vi "rename tag.vi"(7 "owner ID":string, 8 "error in":errorcluster, 9 "new name":string, 10 "old name":string, 11 "engine configuration in":refnum<class "engine configuration.lvclass">) -> (0 "error out":errorcluster, 3 "engine configuration out":refnum<class "engine configuration.lvclass">)   [LabVIEW 2013, in "engine configuration.lvclass"]
doc: "This function is used to rename a tag. If a tag claims to have an owner, only that owner is allowed to modify the tag name."
uses:
  engine configuration.lvclass
  <vilib>/NI/Tag Bus/tag/tag descriptor.lvclass
  <vilib>/NI/Tag Bus/tag/tag descriptor.lvclass/tag descriptor.ctl
  engine configuration.lvclass/engine configuration.ctl
  <vilib>/NI/Configuration Framework/NISE_CEF_TreeControl.lvlib
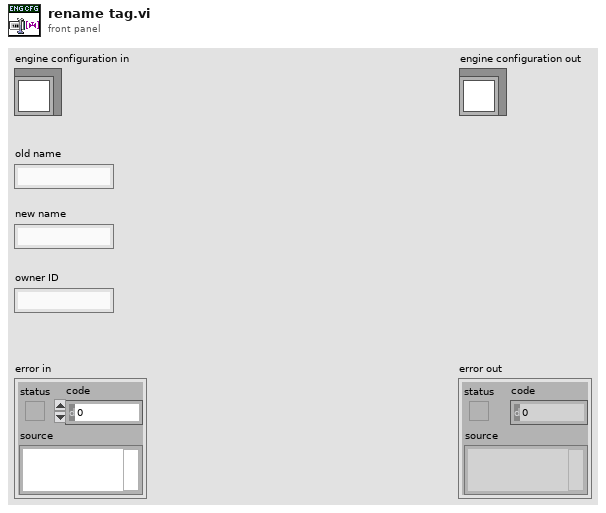
[diagram p1: front panel]
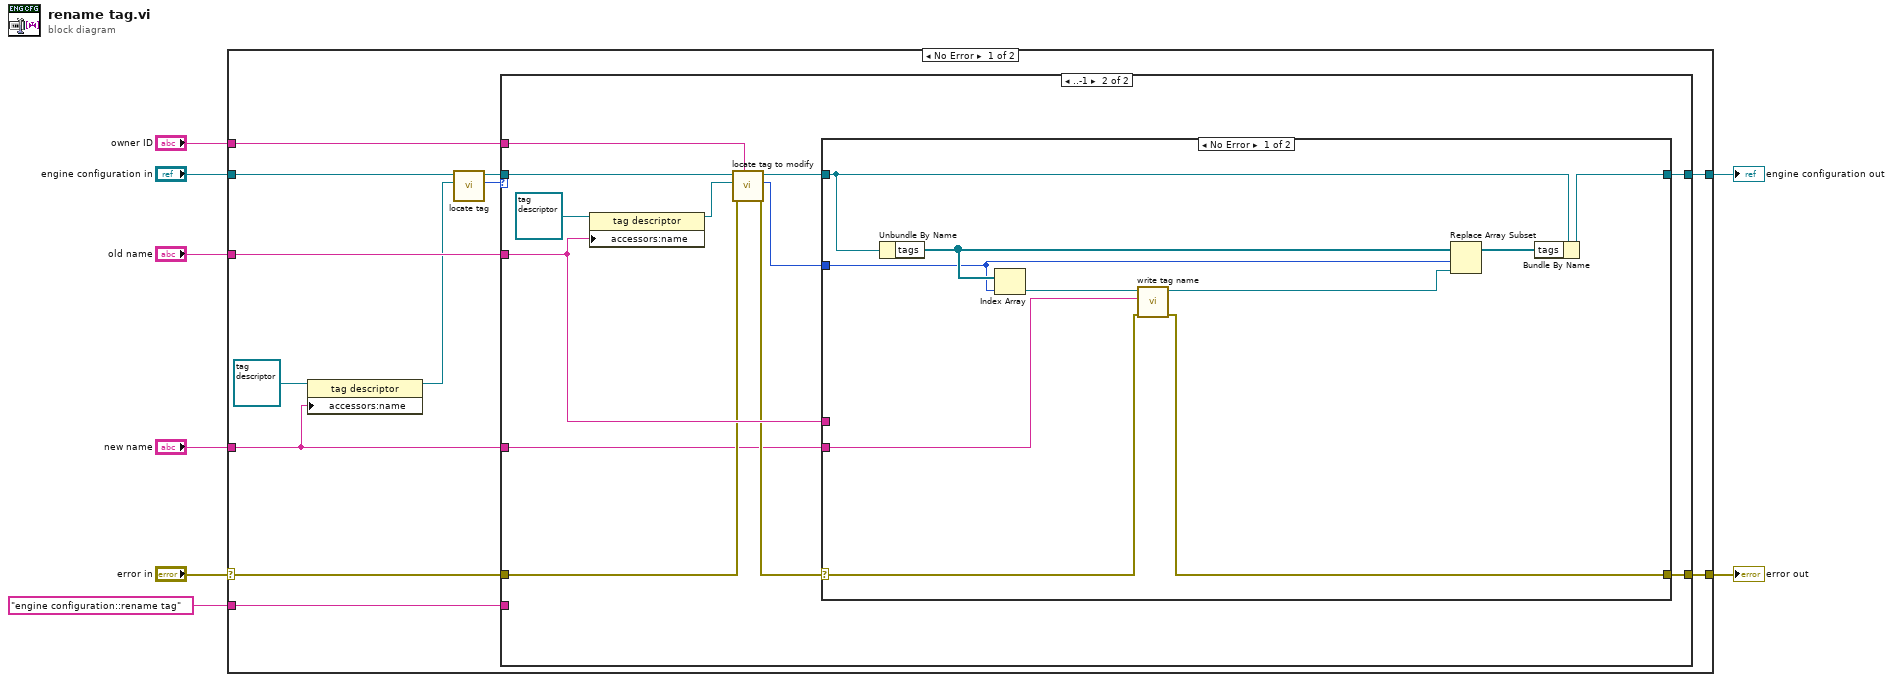
[diagram p0: block diagram]
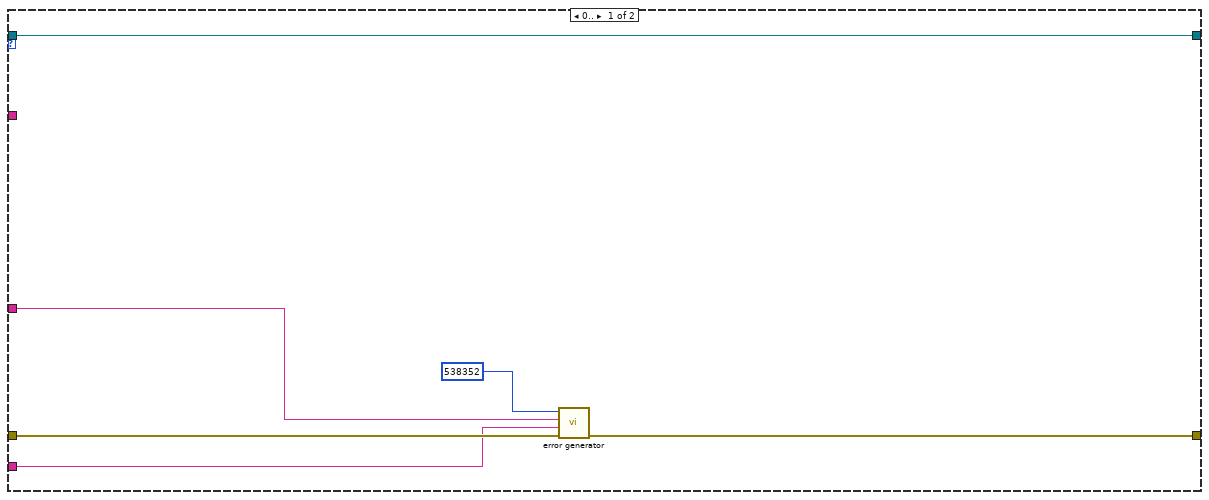
[diagram p2: hidden frame]
diagram:
  n1 = case shown="No Error" "error in" {
    selector: "error in" -> [w16 w52]
    tunnel: [w20 w52] -> w7
    tunnel: [w19 w51] -> w5
    tunnel: "engine configuration in" -> [w15 w51]
    tunnel: "old name" -> [w18 _]
    tunnel: "new name" -> [w12 _]
    tunnel: "owner ID" -> [w17 _]
    tunnel: "engine configuration::rename tag" ("source") -> [w9 _]
    frame No Error {
      n2 = property class="tag descriptor"(reference=refnum<class "tag descriptor.lvclass"> refnum ("tag descriptor"), "accessors:name"=w12) -> (reference out=w11:refnum<class "tag descriptor.lvclass">)  [unwired: 1 in, 1 out]
      n3 = call "locate tag.vi"("tag descriptor"=w11, "engine configuration in"=w15) -> ("index"=w10:i32, "engine configuration out"=w14:refnum<class "engine configuration.lvclass">)  [unwired: 8 in]
      n4 = case shown="..-1" w10 {
        tunnel: [w24 w37] -> w20
        tunnel: [w26 w36] -> w19
        tunnel: w18 -> [_ w35]
        tunnel: w17 -> [_ w33]
        tunnel: w16 -> [w25 w31]
        tunnel: w14 -> [w26 w28]
        tunnel: w12 -> [w23 w27]
        tunnel: w9 -> [w21 _]
        frame 0.. {
          n5 = call <vilib>:"error generator.vi"("error in"=w25, "source"=w21, "append error message"=w23, "error code (0)"=538352) -> ("error out"=w24:errorcluster)  [unwired: 5 in]
        }
        frame ..-1 {
          n6 = property class="tag descriptor"(reference=refnum<class "tag descriptor.lvclass"> refnum ("tag descriptor"), "accessors:name"=w35) -> (reference out=w32:refnum<class "tag descriptor.lvclass">)  [unwired: 1 in, 1 out]
          n7 = call "locate tag to modify.vi"("owner ID"=w33, "error in"=w31, "tag descriptor"=w32, "engine configuration in"=w28) -> ("error out"=w30:errorcluster, "index"=w29:i32, "engine configuration out"=w34:refnum<class "engine configuration.lvclass">)  [unwired: 5 in]
          n8 = case shown="No Error" w30 {
            selector: w30 -> [w41 w49]
            tunnel: [w40 w49] -> w37
            tunnel: w34 -> [w45 w50]
            tunnel: [w46 w50] -> w36
            tunnel: w27 -> [w39 _]
            tunnel: w35 -> [_ _]
            tunnel: w29 -> [w44 _]
            frame No Error {
              n9 = Unbundle By Name(w45) -> ("tags"=w48:refnum<class "tag descriptor.lvclass">[])
              n10 = Index Array(array=w48, index=w44) -> (element=w43:refnum<class "tag descriptor.lvclass">)
              n11 = call <vilib>:"write tag name.vi"("error in"=w41, "name"=w39, "system tag in"=w43) -> ("error out"=w40:errorcluster, "system tag out"=w42:refnum<class "tag descriptor.lvclass">)  [unwired: 7 in]
              n12 = Replace Array Subset(array=w48, new element=w42, index=w44) -> (w47:refnum<class "tag descriptor.lvclass">[])
              n13 = Bundle By Name(cluster=w45, "tags"=w47) -> (w46:refnum<class "engine configuration.lvclass">)
            }
            frame Error {
            }
          }
        }
      }
    }
    frame Error {
    }
  }
  "error out" <- w7
  "engine configuration out" <- w5
